vi "Get Max Profile Size.vi"(4 "Batch On-Off":bool) -> (1 "Profile Size":u32)   [LabVIEW 2014, in "Keyence LJ-V7000.lvlib"]
uses:
  Keyence LJ-V7000.lvlib
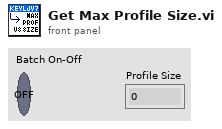
[diagram p1: front panel]
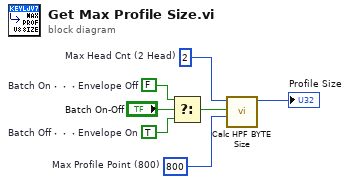
[diagram p0: block diagram]
diagram:
  w4 = TRUE  # Batch Off・・・Envelope On
  w6 = u16 800  # Max Profile Point (800)
  w3 = FALSE  # Batch On・・・Envelope Off
  w7 = u8 2  # Max Head Cnt (2 Head)
  n1 = Select(t=w3, s="Batch On-Off", f=w4) -> (s? t:f=w2:bool)
  n2 = call "Calc HPF BYTE Size.vi"("Profile Data Point"=w6, "Envelope"=w2, "Profile Cnt"=w7) -> ("Profile Size"=→"Profile Size":u32)  [unwired: 8 in]
